vi "Test_DelayGenerator.vi"() -> ()   [LabVIEW 2009]
uses:
  Controls/Baseline.ctl
  Controls/SiteInformation.ctl
  Controls/StarAstrometricEntry.ctl
panel:
  in  "Time Stamp":timestamp
  in  "cat_entry":T1 {"dec" format="%.6g"; "ra" format="%.6g"}
  out "Error":dbl[unit]
  in  "dt":dbl=1.0
  out "Delay Rate (diff)":dbl[unit]
  out "Delay Rate":dbl[unit]
  out "Delay":dbl[unit]
  in  "site_info":T2 {"longitude" format="%_10g"; "latitude" format="%_10g"}
  in  "Baseline":T3 {"Up" format="%.6g"; "North" format="%.6g"; "East" format="%.6g"}
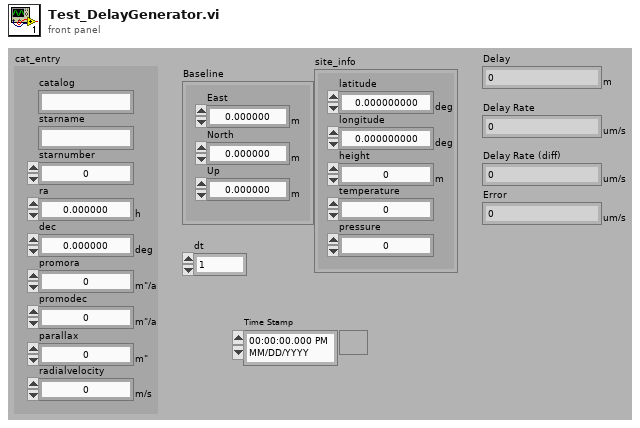
[diagram p1: front panel]
types:
  T1 = typedef "StarAstrometricEntry.ctl" = cluster{"catalog":string, "starname":string, "starnumber":i32, "ra":dbl[unit], "dec":dbl[unit], "promora":dbl[unit], "promodec":dbl[unit], "parallax":dbl[unit], "radialvelocity":dbl[unit]}
  T2 = typedef "SiteInformation.ctl" = cluster{"latitude":dbl[unit], "longitude":dbl[unit], "height":dbl[unit], "temperature":dbl, "pressure":dbl}
  T3 = typedef "Baseline.ctl" = cluster{"East":dbl[unit], "North":dbl[unit], "Up":dbl[unit]}
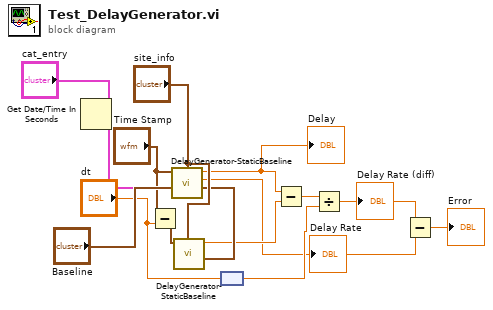
[diagram p0: block diagram]
diagram:
  n1 = Get Date/Time In Seconds() -> ()  [unwired: 1 out]
  n2 = Subtract(x="Time Stamp", y="dt") -> (x-y=w10:timestamp)
  n3 = call "DelayGenerator-StaticBaseline.vi"("site_info"="site_info", "Time Stamp"="Time Stamp", "Baseline"="Baseline", "cat_entry"="cat_entry") -> ("Delay"=w9:dbl[unit], "Delay Rate"=w3:dbl[unit])  [unwired: 3 in, 1 out]
  "Delay" <- w9
  "Delay Rate" <- w3
  n4 = call "DelayGenerator-StaticBaseline.vi"("site_info"="site_info", "Time Stamp"=w10, "Baseline"="Baseline") -> ("Delay"=w8:dbl[unit])  [unwired: 4 in, 2 out]
  n5 = node("dt") -> (w6:dbl[unit])
  n6 = Subtract(x=w9, y=w8) -> (x-y=w7:dbl[unit])
  n7 = Divide(x=w7, y=w6) -> (x/y=w4:dbl[unit])
  "Delay Rate (diff)" <- w4
  n8 = Subtract(x=w4, y=w3) -> (x-y=→"Error":dbl[unit])
